vi "VI-Build Project (Full) Dialog.vi"() -> ()   [LabVIEW 2020]
uses:
  <vilib>/Utility/error.llb/DialogType.ctl
  <vilib>/AppBuilder/AB_API_Simple/Build (path).vi
  <vilib>/AppBuilder/AB_API_Simple/NI_App_Builder_API.lvlib
panel:
  out "log":string
  out "Slide":u8(slide) scale=0.0..100.0
  out "abort":bool
  in  "Quit":bool
  # "Build"
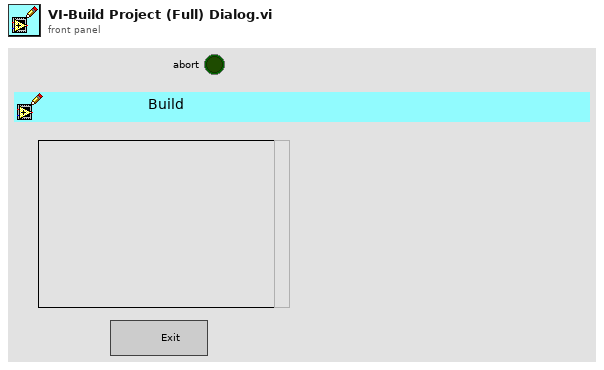
[diagram p1: front panel]
types:
  T1 = typedef "DialogType.ctl" = u16
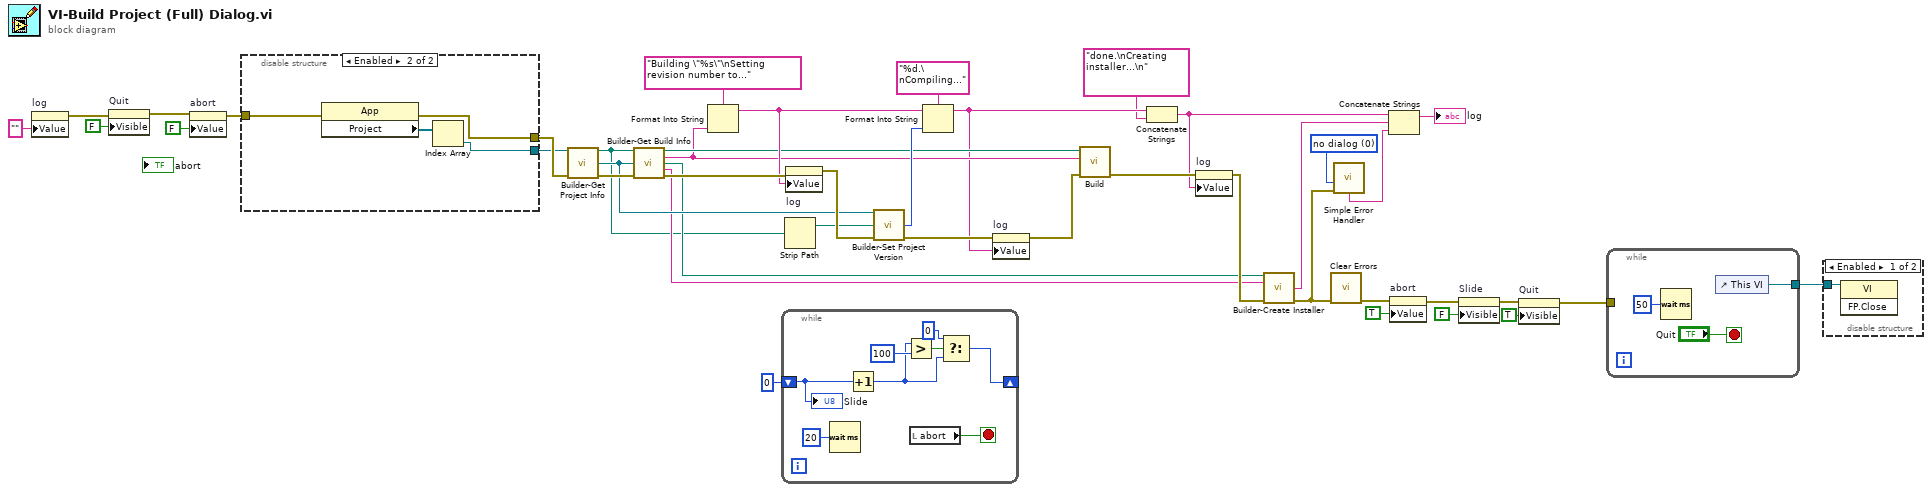
[diagram p0: block diagram]
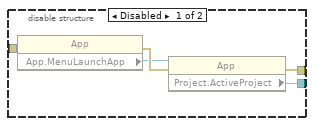
[diagram p3: hidden frame]
diagram:
  w13 = T1 0 items=["no dialog", "OK message", "continue or stop message", "OK message + warnings", "continue/stop + warnings"] ("type of dialog (OK msg:1)")
  n1 = property on="log" class="Str"("Value"="" ("log")) -> (error out=w35:errorcluster)  [unwired: 2 in, 1 out]
  n2 = property on="Quit" class="Bool"(error in=w35, "Visible"=FALSE) -> (error out=w39:errorcluster)  [unwired: 1 in, 1 out]
  n3 = property on="abort" class="Bool (strict)"(error in=w39, "Value"=FALSE ("abort")) -> (error out=w41:errorcluster)  [unwired: 1 in, 1 out]
  n4 = disable-structure shown="Enabled" {
    disable-tunnel: w41 -> [w46 w51]
    disable-tunnel: [w45 w49] -> w37
    disable-tunnel: [w44 w50] -> w36
    frame Disabled {
      n5 = property class="App"(error in=w46) -> (error out=w48:errorcluster, "App.MenuLaunchApp"=w47:refnum<vi>)  [unwired: 1 in, 1 out]
      n6 = property class="App"(reference=w47, error in=w48) -> (error out=w45:errorcluster, "Project.ActiveProject"=w44:refnum<vi>)  [unwired: 1 out]
    }
    frame Enabled {
      n7 = property class="App"(error in=w51) -> (error out=w49:errorcluster, "Project"=w52:refnum<vi>[])  [unwired: 1 in, 1 out]
      n8 = Index Array(array=w52) -> (element=w50:refnum<vi>)  [unwired: 1 in]
    }
  }
  n9 = call "Builder-Get Project Info.vi"("Project ref"=w36, "error in (no error)"=w37) -> ("Project Path"=w2:path, "ProjectItem"=w30:refnum<vi>, "error out"=w33:errorcluster)  [unwired: 11 in]
  n10 = call "Builder-Get Build Info.vi"("Project Path in"=w2, "Project Item"=w30, "error in (no error)"=w33) -> ("Project Path out"=w25:path, "Build Spec Name"=w23:string, "Exe Path"=w17:path, "Product Name"=w18:string, "error out"=w32:errorcluster)  [unwired: 8 in]
  n11 = Format Into String(format string="Building \"%s\"\nSetting revision number to...", w23) -> (resulting string=w29:string)  [unwired: 2 in, 1 out]
  n12 = while {
    shift-right: [w58] -> _
    shift-left: 0 -> [w55]
    stop <- w53 stop-if-true
    n13 = Wait (ms)(milliseconds to wait=u32 20) -> ()  [unwired: 1 out]
    n14 = Increment(x=w55) -> (x+1=w57:i32)
    n15 = Greater?(x=w57, y=100) -> (0:w59:bool)
    n16 = local read "abort"() -> (w53:bool)
    n17 = Select(t=0, s=w59, f=w57) -> (s? t:f=w58:i32)
    "Slide" <- w55
  }
  n18 = Strip Path(path=w2) -> (stripped path=w1:path)  [unwired: 1 out]
  n19 = property on="log" class="Str"(error in=w32, "Value"=w29) -> (error out=w31:errorcluster)  [unwired: 1 in, 1 out]
  n20 = call "Builder-Set Project Version.vi"("ProjectItem in"=w30, "Path"=w1, "error in (no error)"=w31) -> ("revision"=w27:i32, "error out"=w26:errorcluster)  [unwired: 10 in, 1 out]
  n21 = Format Into String(format string="%d.\nCompiling...", initial string=w29, w27) -> (resulting string=w22:string)  [unwired: 1 in, 1 out]
  n22 = property on="log" class="Str"(error in=w26, "Value"=w22) -> (error out=w24:errorcluster)  [unwired: 1 in, 1 out]
  n23 = call-poly <vilib>:"Build.vi"("error in (no error)"=w24, "Name of build specification (if empty: build all)"=w23, "Path to project"=w25) -> ("error out"=w20:errorcluster)  [unwired: 7 in, 1 out]
  n24 = Concatenate Strings(w22, "done.\nCreating installer...\n" ("format string")) -> (w16:string)
  n25 = property on="log" class="Str"(error in=w20, "Value"=w16) -> (error out=w19:errorcluster)  [unwired: 1 in, 1 out]
  n26 = call "Builder-Create Installer.vi"("Exe Path"=w17, "Product Name"=w18, "error in (no error)"=w19) -> ("standard error"=w15:string, "error out"=w10:errorcluster)  [unwired: 11 in]
  n27 = call <vilib>:"Clear Errors.vi"("error in (no error)"=w10) -> ("error out"=w9:errorcluster)  [unwired: 5 in, 1 out]
  n28 = call <vilib>:"Simple Error Handler.vi"("type of dialog (OK msg:1)"=w13, "error in (no error)"=w10) -> ("message"=w12:string)  [unwired: 3 in, 4 out]
  n29 = Concatenate Strings(w16, w15, w12) -> (→"log":string)
  n30 = property on="abort" class="Bool (strict)"(error in=w9, "Value"=TRUE ("abort")) -> (error out=w8:errorcluster)  [unwired: 1 in, 1 out]
  n31 = property on="Slide" class="Slide (strict)"(error in=w8, "Visible"=FALSE) -> (error out=w6:errorcluster)  [unwired: 1 in, 1 out]
  n32 = property on="Quit" class="Bool"(error in=w6, "Visible"=TRUE) -> (error out=w3:errorcluster)  [unwired: 1 in, 1 out]
  n33 = while {
    tunnel: [w62] -> w4
    tunnel: w3 -> [_]
    stop <- "Quit" stop-if-true
    n34 = Wait (ms)(milliseconds to wait=u32 50) -> ()  [unwired: 1 out]
    n35 = control-ref of="This VI"() -> (w62:refnum<vi>)
  }
  n36 = disable-structure shown="Enabled" {
    disable-tunnel: w4 -> [w64 _]
    frame Enabled {
      n37 = invoke class="VI" method="FP.Close"(reference=w64) -> ()  [unwired: 2 in, 3 out]
    }
    frame Disabled {
    }
  }
